vi "ContRunPre.vi"(5 "line trig":bool=TRUE, 8 "error in":errorcluster, 11 "Pre Pulse In":T1) -> (0 "error out":errorcluster)   [LabVIEW 2019]
uses:
  PulseControl.ctl
  Compiler/Params.ctl
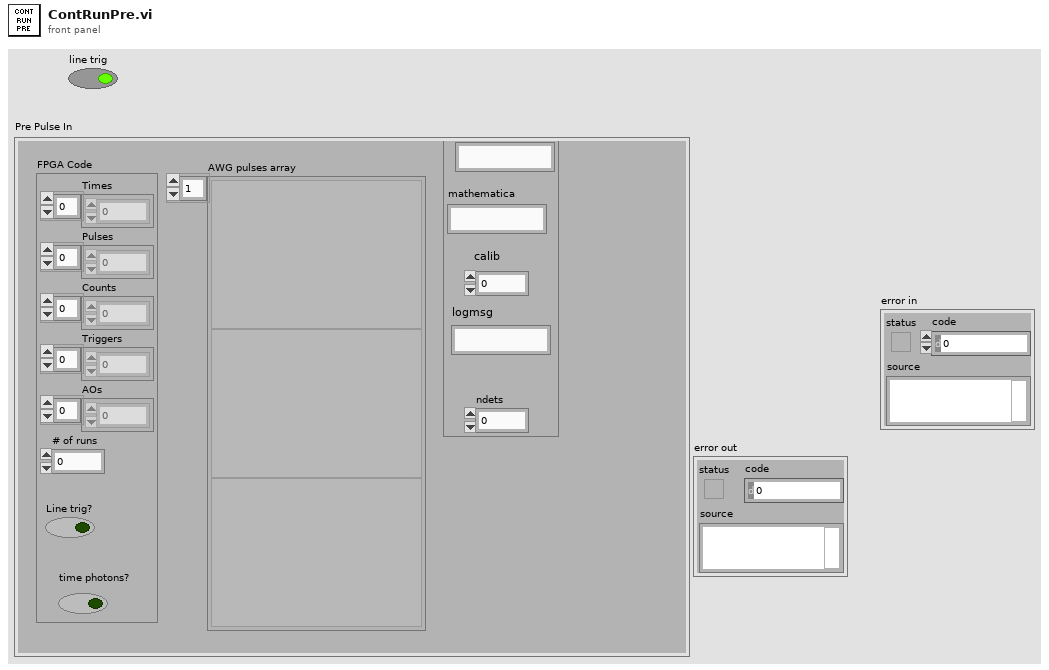
[diagram p1: front panel]
types:
  T1 = typedef "PulseControl.ctl" = cluster{"FPGA Code":cluster{"Times":u32[], "Pulses":u64[], "Counts":u8[], "Triggers":u8[], "AOs":u8[], "# of runs":i32, "Line trig?":bool, "time photons?":bool}, "AWG pulses array":variant[], "Params":T2}
  T2 = typedef "Params.ctl" = cluster{"steps":i16, "runs":i16, "comment":string, "mathematica":string, "calib":i8, "logmsg":string, "ndets":i16}
  T3 = cluster{"Times":u32[], "Pulses":u64[], "Counts":u8[], "Triggers":u8[], "AOs":u8[], "# of runs":i32, "Line trig?":bool, "time photons?":bool}
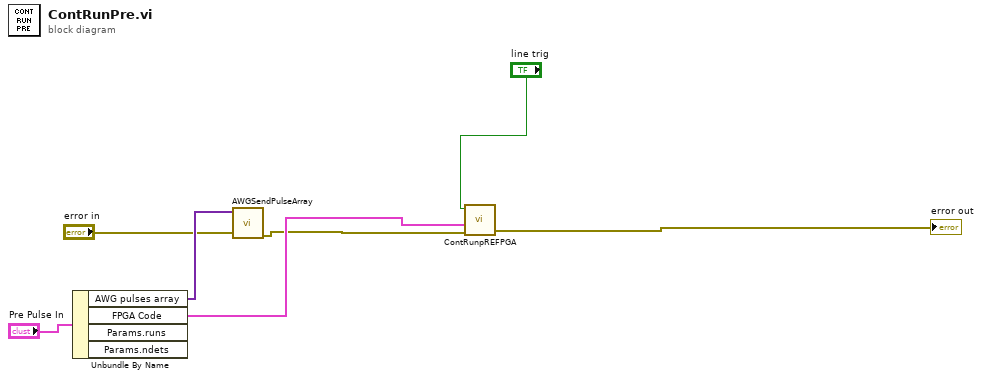
[diagram p0: block diagram]
diagram:
  n1 = Unbundle By Name("Pre Pulse In") -> ("AWG pulses array"=w4:variant[], "FPGA Code"=w6:T3)  [unwired: 2 out]
  n2 = call "AWGSendPulseArray.vi"("error in (no error)"="error in", "AWG pulses array"=w4) -> ("error out"=w2:errorcluster)  [unwired: 9 in]
  n3 = call "ContRunpREFPGA.vi"("error in"=w2, "Cluster"=w6, "Line trig?"="line trig") -> ("error out"=→"error out":errorcluster)  [unwired: 1 in, 2 out]
